vi "Graham Scan Cross Product.vi"(1 "B":T1, 2 "A":T1) -> (0 "C":i32)   [LabVIEW 2018]
uses:
  Graham Scan Point.ctl
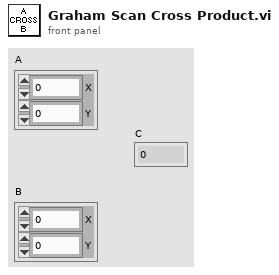
[diagram p1: front panel]
types:
  T1 = typedef "Graham Scan Point.ctl" = cluster{"X":i32, "Y":i32}
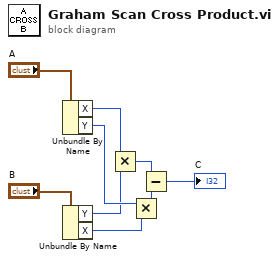
[diagram p0: block diagram]
diagram:
  n1 = Unbundle By Name("A") -> ("X"=w7:i32, "Y"=w3:i32)
  n2 = Unbundle By Name("B") -> ("Y"=w1:i32, "X"=w2:i32)
  n3 = Multiply(x=w7, y=w1) -> (x*y=w6:i32)
  n4 = Multiply(x=w3, y=w2) -> (x*y=w5:i32)
  n5 = Subtract(x=w6, y=w5) -> (x-y=→"C":i32)
